vi "wd_create (Time).vi"(7 "data":timestamp[](array[timestamp]), 8 "error in (no error)":errorcluster, 9 "data type":T1, 11 "meta in":T2={"TargetFile"=path "", "StreamMode"=enum."File", "Append?"=FALSE, "ChunkSize"=0, "TimeColumnMode"=enum."Empty", "TimestampFormat"="", "AbsoluteTime?"=FALSE, "FileAttribute "={"Creator"="", "Title"="", "SheetName"=""}, "Column"=[], "FileRef"=refnum, "MemoryRef"=[], "RecordInfo"=[], " ChannelPreviousInfo"=[], "ChannelFirstRecord"=[], "PredefinedFormattedValueLength"=20, "DiskTemplate"={"XMLRef"=[refnum, refnum, refnum, refnum, refnum, refnum], "ZipPath"=path "", "MetaFile"={"Ref"=refnum, "NextRow"=0, "NextPosition"=0, "Block"=[]}, "TempFolder"=path ""}}) -> (0 "error out":errorcluster, 3 "meta out":T2={"TargetFile"=path "", "StreamMode"=enum."File", "Append?"=FALSE, "ChunkSize"=0, "TimeColumnMode"=enum."Empty", "TimestampFormat"="", "AbsoluteTime?"=FALSE, "FileAttribute "={"Creator"="", "Title"="", "SheetName"=""}, "Column"=[], "FileRef"=refnum, "MemoryRef"=[], "RecordInfo"=[], " ChannelPreviousInfo"=[], "ChannelFirstRecord"=[], "PredefinedFormattedValueLength"=20, "DiskTemplate"={"XMLRef"=[refnum, refnum, refnum, refnum, refnum, refnum], "ZipPath"=path "", "MetaFile"={"Ref"=refnum, "NextRow"=0, "NextPosition"=0, "Block"=[]}, "TempFolder"=path ""}})   [LabVIEW 2017, in "NI_ExcelFile.lvlib"]
uses:
  <vilib>/express/express shared/NI_ExcelFile/NI_ExcelFile.lvlib
  <vilib>/express/express shared/NI_ExcelFile/Ctrls/MainData.ctl
  <vilib>/express/express shared/NI_ExcelFile/Ctrls/StreamMode.ctl
  <vilib>/express/express shared/NI_ExcelFile/Ctrls/TimeColumnMode.ctl
  <vilib>/express/express shared/NI_ExcelFile/Ctrls/FileAttribute.ctl
  <vilib>/express/express shared/NI_ExcelFile/Ctrls/Columns.ctl
  <vilib>/express/express shared/NI_ExcelFile/Ctrls/ColumnInfo.ctl
  <vilib>/express/express shared/NI_ExcelFile/Ctrls/DataType.ctl
  <vilib>/express/express shared/NI_ExcelFile/Ctrls/wd_recordInfo.ctl
  <vilib>/express/express shared/NI_ExcelFile/Ctrls/disk_TemplateFile.ctl
  <vilib>/express/express shared/NI_ExcelFile/Ctrls/meta_file.ctl
  <vilib>/express/express shared/NI_ExcelFile/Ctrls/meta_Block.ctl
  <vilib>/express/express shared/NI_ExcelFile/Ctrls/meta_BlockType.ctl
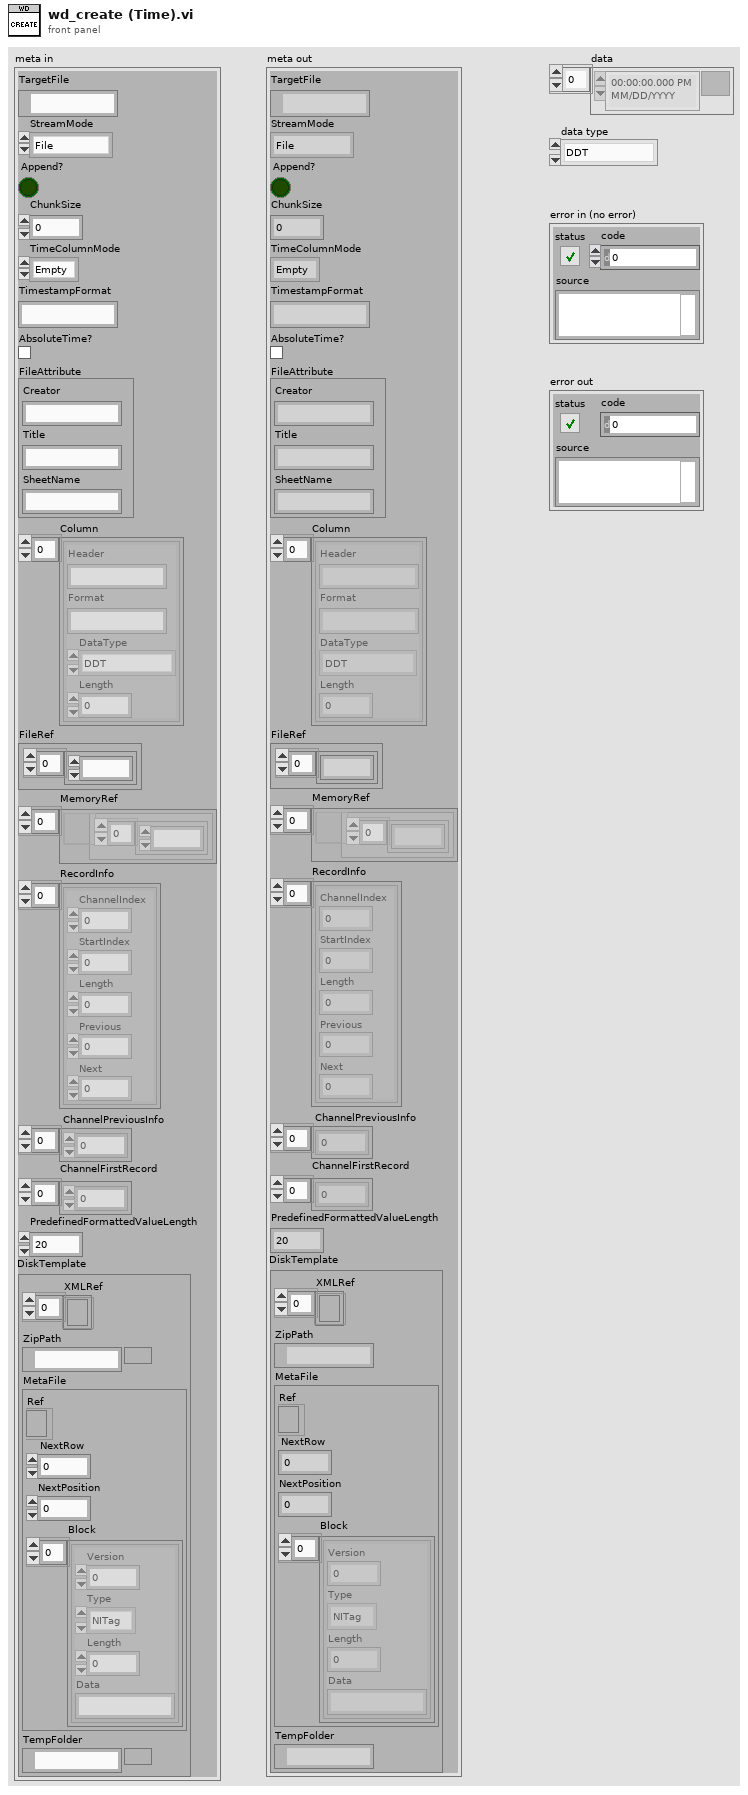
[diagram p1: front panel]
types:
  T1 = typedef "NI_ExcelFile.lvlib/DataType.ctl" = enum16{"DDT", "WFM", "Array of STR", "Array of DBL", "Array of I8", "Array of I16", "Array of I32", "Array of I64", "Array of SGL", "Array of U8", "Array of U16", "Array of U32", "Array of U64", "Array of Time"}
  T2 = typedef "NI_ExcelFile.lvlib/MainData.ctl" = cluster{"TargetFile":path, "StreamMode":T3, "Append?":bool, "ChunkSize":u64, "TimeColumnMode":T4, "TimestampFormat":string, "AbsoluteTime?":bool, "FileAttribute ":T5, "Column":T6, "FileRef":refnum<k1>, "MemoryRef":refnum<data-value>[], "RecordInfo":T8[], " ChannelPreviousInfo":u32[], "ChannelFirstRecord":u32[], "PredefinedFormattedValueLength":i64, "DiskTemplate":T9}
  T3 = typedef "NI_ExcelFile.lvlib/StreamMode.ctl" = enum16{"File", "Memory"}
  T4 = typedef "NI_ExcelFile.lvlib/TimeColumnMode.ctl" = enum16{"Empty", "OnePerCh", "One"}
  T5 = typedef "NI_ExcelFile.lvlib/FileAttribute.ctl" = cluster{"Creator":string, "Title":string, "SheetName":string}
  T6 = typedef "NI_ExcelFile.lvlib/Columns.ctl" = T7[]
  T7 = typedef "NI_ExcelFile.lvlib/ColumnInfo.ctl" = cluster{"Header":string, "Format":string, "DataType":T1, "Length":u64}
  T8 = typedef "NI_ExcelFile.lvlib/wd_recordInfo.ctl" = cluster{"ChannelIndex":u32, "StartIndex":u64, "Length":u64, "Previous":i32, "Next":i32}
  T9 = typedef "NI_ExcelFile.lvlib/disk_TemplateFile.ctl" = cluster{"XMLRef":refnum<file>[], "ZipPath":path, "MetaFile":T10, "TempFolder":path}
  T10 = typedef "NI_ExcelFile.lvlib/meta_file.ctl" = cluster{"Ref":refnum<file>, "NextRow":i32, "NextPosition":i64, "Block":T11[]}
  T11 = typedef "NI_ExcelFile.lvlib/meta_Block.ctl" = cluster{"Version":u16, "Type":T12, "Length":i32, "Data":string}
  T12 = typedef "NI_ExcelFile.lvlib/meta_BlockType.ctl" = enum16{"NITag", "File", "Column"}
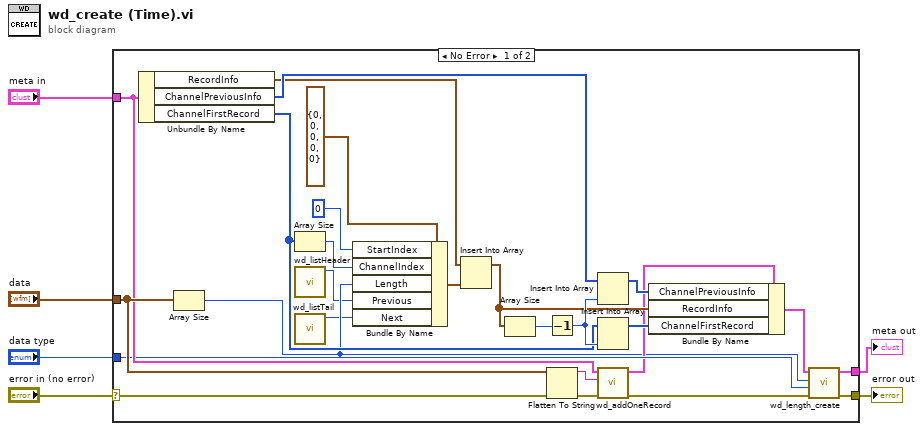
[diagram p0: block diagram]
diagram:
  n1 = case shown="No Error" "error in (no error)" {
    selector: "error in (no error)" -> [w22 w33]
    tunnel: "data type" -> [w19 _]
    tunnel: [w16 w34] -> w5
    tunnel: "meta in" -> [w20 w34]
    tunnel: "data" -> [w24 _]
    tunnel: [w14 w33] -> w1
    frame No Error {
      n2 = Unbundle By Name(w20) -> ("RecordInfo"=w26:T8[], "ChannelPreviousInfo"=w27:u32[], "ChannelFirstRecord"=w25:u32[])
      n3 = Array Size(array=w24) -> (size(s)=w11:i32)
      n4 = Array Size(array=w25) -> (size(s)=w9:i32)
      n5 = call <vilib>:"wd_listHeader.vi"() -> ("list header"=w8:i32)  [unwired: 11 in]
      n6 = call <vilib>:"wd_listTail.vi"() -> ("list tail"=w7:i32)  [unwired: 11 in]
      n7 = Bundle By Name(cluster=T8 {"ChannelIndex"=0, "StartIndex"=0, "Length"=0, "Previous"=0, "Next"=0} ("Channel Info"), "StartIndex"=u64 0 ("Start Index"), "ChannelIndex"=w9, "Length"=w11, "Previous"=w8, "Next"=w7) -> (w12:T8)
      n8 = Insert Into Array(array=w26, new element=w12) -> (w30:T8[])  [unwired: 1 in]
      n9 = Array Size(array=w30) -> (size(s)=w29:i32)
      n10 = Decrement(x=w29) -> (x-1=w31:i32)
      n11 = Flatten To String(anything=w24, error in (no error)=w22) -> (data string=w23:string, error out=w21:errorcluster)  [unwired: 2 in, 1 out]
      n12 = Insert Into Array(array=w27, new element=w31) -> (w28:u32[])  [unwired: 1 in]
      n13 = Insert Into Array(array=w25, new element=w31) -> (w32:u32[])  [unwired: 1 in]
      n14 = call <vilib>:"wd_addOneRecord.vi"("error in (no error)"=w21, "data"=w23, "meta in"=w20) -> ("error out"=w15:errorcluster, "meta out"=w18:T2)  [unwired: 7 in]
      n15 = Bundle By Name(cluster=w18, "ChannelPreviousInfo"=w28, "RecordInfo"=w30, "ChannelFirstRecord"=w32) -> (w17:T2)
      n16 = call <vilib>:"wd_length_create.vi"("error in (no error)"=w15, "data type"=w19, "size"=w11, "meta in"=w17) -> ("error out"=w14:errorcluster, "meta out"=w16:T2)  [unwired: 6 in]
    }
    frame Error {
    }
  }
  "error out" <- w1
  "meta out" <- w5
